vi "CheckUserAndPwd.vi"(6 "TableName(\"\")":string, 8 "error in (no error)":errorcluster, 9 "Pwd(\"\")":string, 10 "Name(\"\")":string, 11 "Login in":refnum<class "Login.lvclass">) -> (0 "error out":errorcluster, 1 "ID('')":string, 2 "Has(False)":bool, 3 "Login out":refnum<class "Login.lvclass">, 4 "ActualName(\"\")":string)   [LabVIEW 2015, in "Login.lvclass"]
uses:
  Login.lvclass
  Login.lvclass/Login.ctl
  API/_Database/Database.lvclass
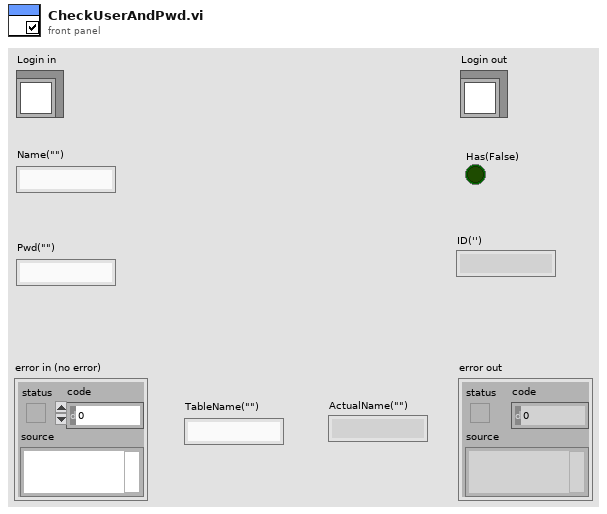
[diagram p1: front panel]
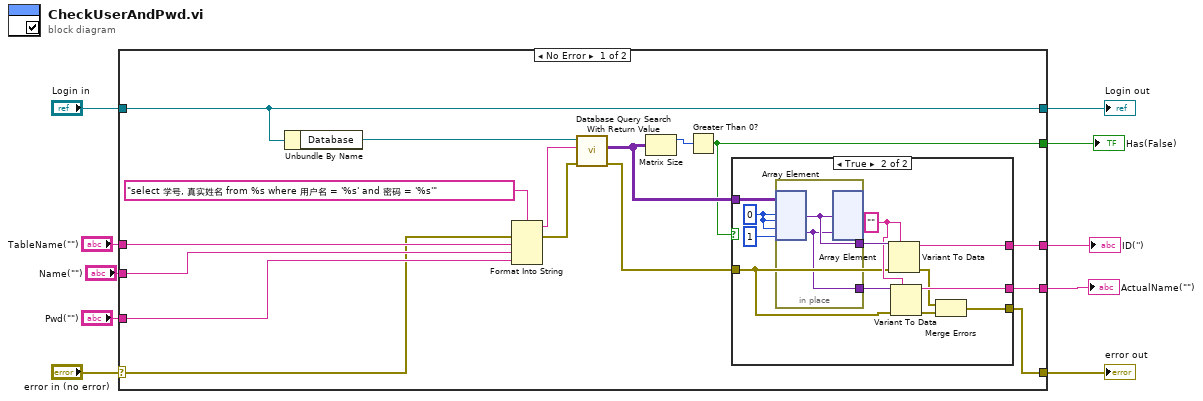
[diagram p0: block diagram]
diagram:
  n1 = case shown="No Error" "error in (no error)" {
    selector: "error in (no error)" -> [w19 w43]
    tunnel: [w14 w43] -> w9
    tunnel: [w26 w42] -> w7
    tunnel: "Login in" -> [w26 w42]
    tunnel: "Name(\"\")" -> [w22 _]
    tunnel: "Pwd(\"\")" -> [w21 _]
    tunnel: "TableName(\"\")" -> [w23 _]
    tunnel: [w12 _] -> w3
    tunnel: [w13 _] -> w2
    tunnel: [w11 _] -> w1
    frame No Error {
      n2 = Unbundle By Name(w26) -> ("Database"=w25:refnum<class "Database.lvclass">)
      n3 = Format Into String(format string="select 学号, 真实姓名 from %s where 用户名 = '%s' and 密码 = '%s'", error in=w19, w23, w22, w21) -> (resulting string=w20:string, error out=w18:errorcluster)  [unwired: 1 in]
      n4 = call "Database Query Search With Return Value.vi"("error in (no error)"=w18, "SQL query"=w20, "object in"=w25) -> ("error out"=w15:errorcluster, "recordset data"=w16:variant[][])  [unwired: 5 in, 2 out]
      n5 = Matrix Size(0:w16) -> (1:w17:i32)  [unwired: 1 out]
      n6 = Greater Than 0?(x=w17) -> (x > 0?=w12:bool)
      n7 = case shown="True" w12 {
        tunnel: w16 -> [_ w39]
        tunnel: w15 -> [w27 w32]
        tunnel: [w27 w28] -> w14
        tunnel: [_ w37] -> w13
        tunnel: [_ w31] -> w11
        frame False {
        }
        frame True {
          w33 = ""
          w36 = 0
          n8 = in-place {
            in-place-border: [w41] -> w38
            in-place-border: [w40] -> w34
            n9 = in-place-array #1(w39, w36, w36, w36, 1) -> (w41:variant, w40:variant)
            n10 = in-place-array #1(w41, w40) -> ()  [unwired: 5 out]
          }
          n11 = Variant To Data(error in=w32, type=w33, Variant=w38) -> (data=w37:string, error out=w29:errorcluster)
          n12 = Variant To Data(error in=w32, type=w33, Variant=w34) -> (data=w31:string, error out=w30:errorcluster)
          n13 = Merge Errors(w29, w30) -> (w28:errorcluster)
        }
      }
    }
    frame Error {
    }
  }
  "error out" <- w9
  "Login out" <- w7
  "Has(False)" <- w3
  "ID('')" <- w2
  "ActualName(\"\")" <- w1
